vi "Get Config From File.vi"(8 "error in (no error)":errorcluster, 11 "XboxController-V in":refnum<class "XboxController-V.lvclass">) -> (0 "error out":errorcluster, 3 "XboxController-V out":refnum<class "XboxController-V.lvclass">)   [LabVIEW 2013]
uses:
  Virtual Systems/XBoxController-V/XboxController-V.lvclass
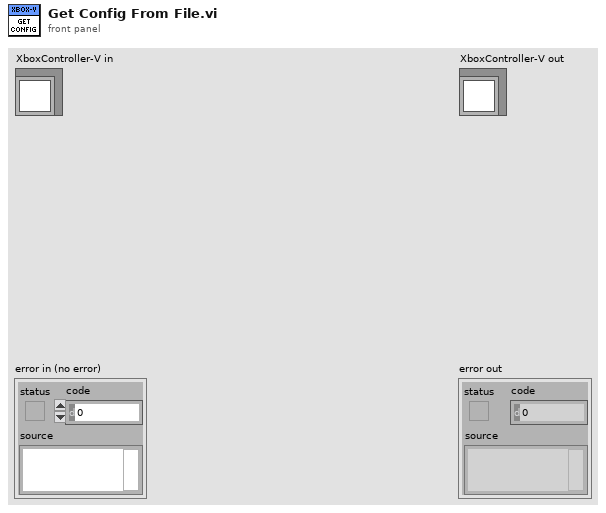
[diagram p1: front panel]
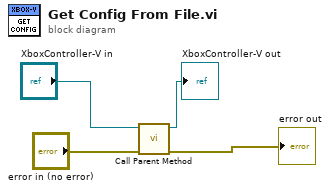
[diagram p0: block diagram]
diagram:
  n1 = call-parent "Call Parent Method"("error in (no error)"="error in (no error)", "System in"="XboxController-V in") -> ("error out"=→"error out":errorcluster, "System out"=→"XboxController-V out":refnum<class "XboxController-V.lvclass">)  [unwired: 7 in, 1 out]
